vi "FPGA_MotorControl.vi"() -> ()   [LabVIEW 2013]
uses:
  <vilib>/Platform/TimedLoop/XDataNode/timing_clust.ctl
  <vilib>/Platform/TimedLoop/XDataNode/nitl_modes.ctl
  <vilib>/Platform/TimedLoop/XDataNode/wakeup.ctl
  <vilib>/rvi/FXPMathLib/FxpDiv/subVIs/nifxpmath_Div_SimConfig.ctl
  <vilib>/rvi/Emulation/niFpgaSctlEmulationGetInTimedLoop.vi
  <vilib>/rvi/Emulation/niFpgaEmulationReportErrorSimple.vi
  <vilib>/rvi/Emulation/niFpgaGetClockAttributes.vi
  <vilib>/rvi/Emulation/niFpgaCriticalErrorInLSC.vi
  GVEncoder.vi
  <vilib>/rvi/eio/common/nirviEmuTemplateMethod_errors.vi
  <vilib>/rvi/Emulation/niFpgaProcessEmulError.vi
  <vilib>/rvi/FXPMathLib/FxpDiv/simVIs/DllFxpDivTemp_sub.vi
  <vilib>/Platform/TimedLoop/XDataNode/XDataNode.xnode
  <vilib>/eio/EIONode/EIONode.xnode
  <vilib>/rvi/FXPMathLib/FxpMul/XNode/nifxpmath_Multiplier.xnode
  <vilib>/rvi/FXPMathLib/FxpDiv/XNode/nifxpmath_Div.xnode
  <vilib>/rvi/Analysis/measure/butterworth/XNode/niFpgaButterworthFilter.xnode
  <vilib>/Platform/TimedLoop/XDataNode/XDNodeRunTimeDep.lvlib
  <vilib>/rvi/FXPMathLib/sim/FxpSim.dll
panel:
  in  "Reset Position 8":bool
  in  "Reset Position 7":bool
  in  "Reset Position 6":bool
  in  "Reset Position 5":bool
  in  "Reset Position 4":bool
  out "EncdSpeed":sgl[](array[numeric])
  out "EncdAngle":sgl[](array[numeric]) format="%#.3f"
  in  "2pi":fxp<+/-,32,10>=6.283185243606567 format="%#_39g"
  in  "EncoderCount":fxp<+,16,16>=2048.0
  in  "Reset Position 3":bool
  in  "Reset Position 2":bool
  in  "Reset Position 1":bool
  in  "AO_Value":sgl[](array[numeric])=[0.0, 0.0, 0.0, 0.0, 0.0, 0.0, 0.0, 0.0]
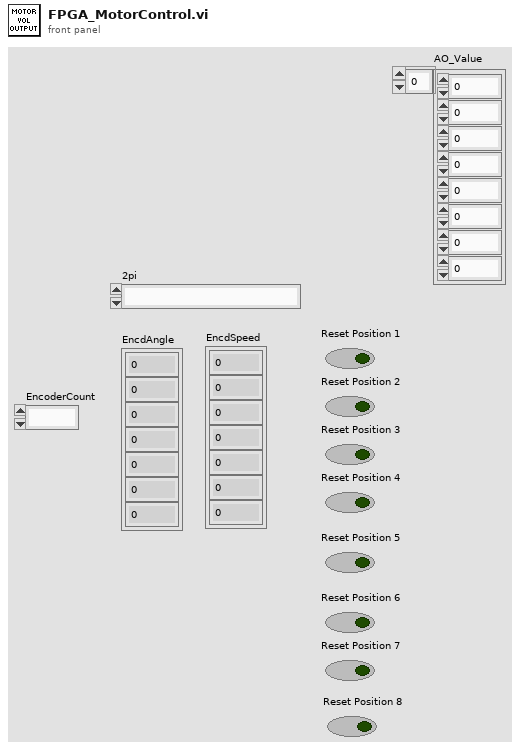
[diagram p1: front panel]
types:
  T1 = typedef "XDNodeRunTimeDep.lvlib/timing_clust.ctl" = cluster{"Expected End [f-1]":u64, "Actual End [f-1]":u64, "Finished Late? [f-1]":bool, "Expected End [i-1]":u64, "Actual End [i-1]":u64, "Finished Late? [i-1]":bool, "Expected Start [i]":u64, "Actual Start [i]":u64, "Expected Start [f]":u64, "Actual Start [f]":u64, "Source Name":string, "Structure Name":string, "Period":i64, "Deadline":i64, "Offset":i64, "Start":i64, "Priority":i32, "Timeout":i32, "Mode":T2, "Wakeup Reason":T3, "Error":errorcluster, "Source Type":string, "Secondary Source Type":string, "Global End Time":u64, "Global Start Time":u64, "Frame Duration":u64, "Iteration Duration":u64, "Assigned CPU":i32, "I/O Scan Engine Mode":u32}
  T2 = typedef "XDNodeRunTimeDep.lvlib/nitl_modes.ctl" = enum32{"No Change", "Process missed periods, maintain original phase", "Discard missed periods, maintain original phase", "Process missed periods, ignore original phase", "Discard missed periods, ignore original phase"}
  T3 = typedef "XDNodeRunTimeDep.lvlib/wakeup.ctl" = enum32{"Normal", "Aborted", "Asynchronous wakeup", "Timing source error", "Timed loop error", "Timeout"}
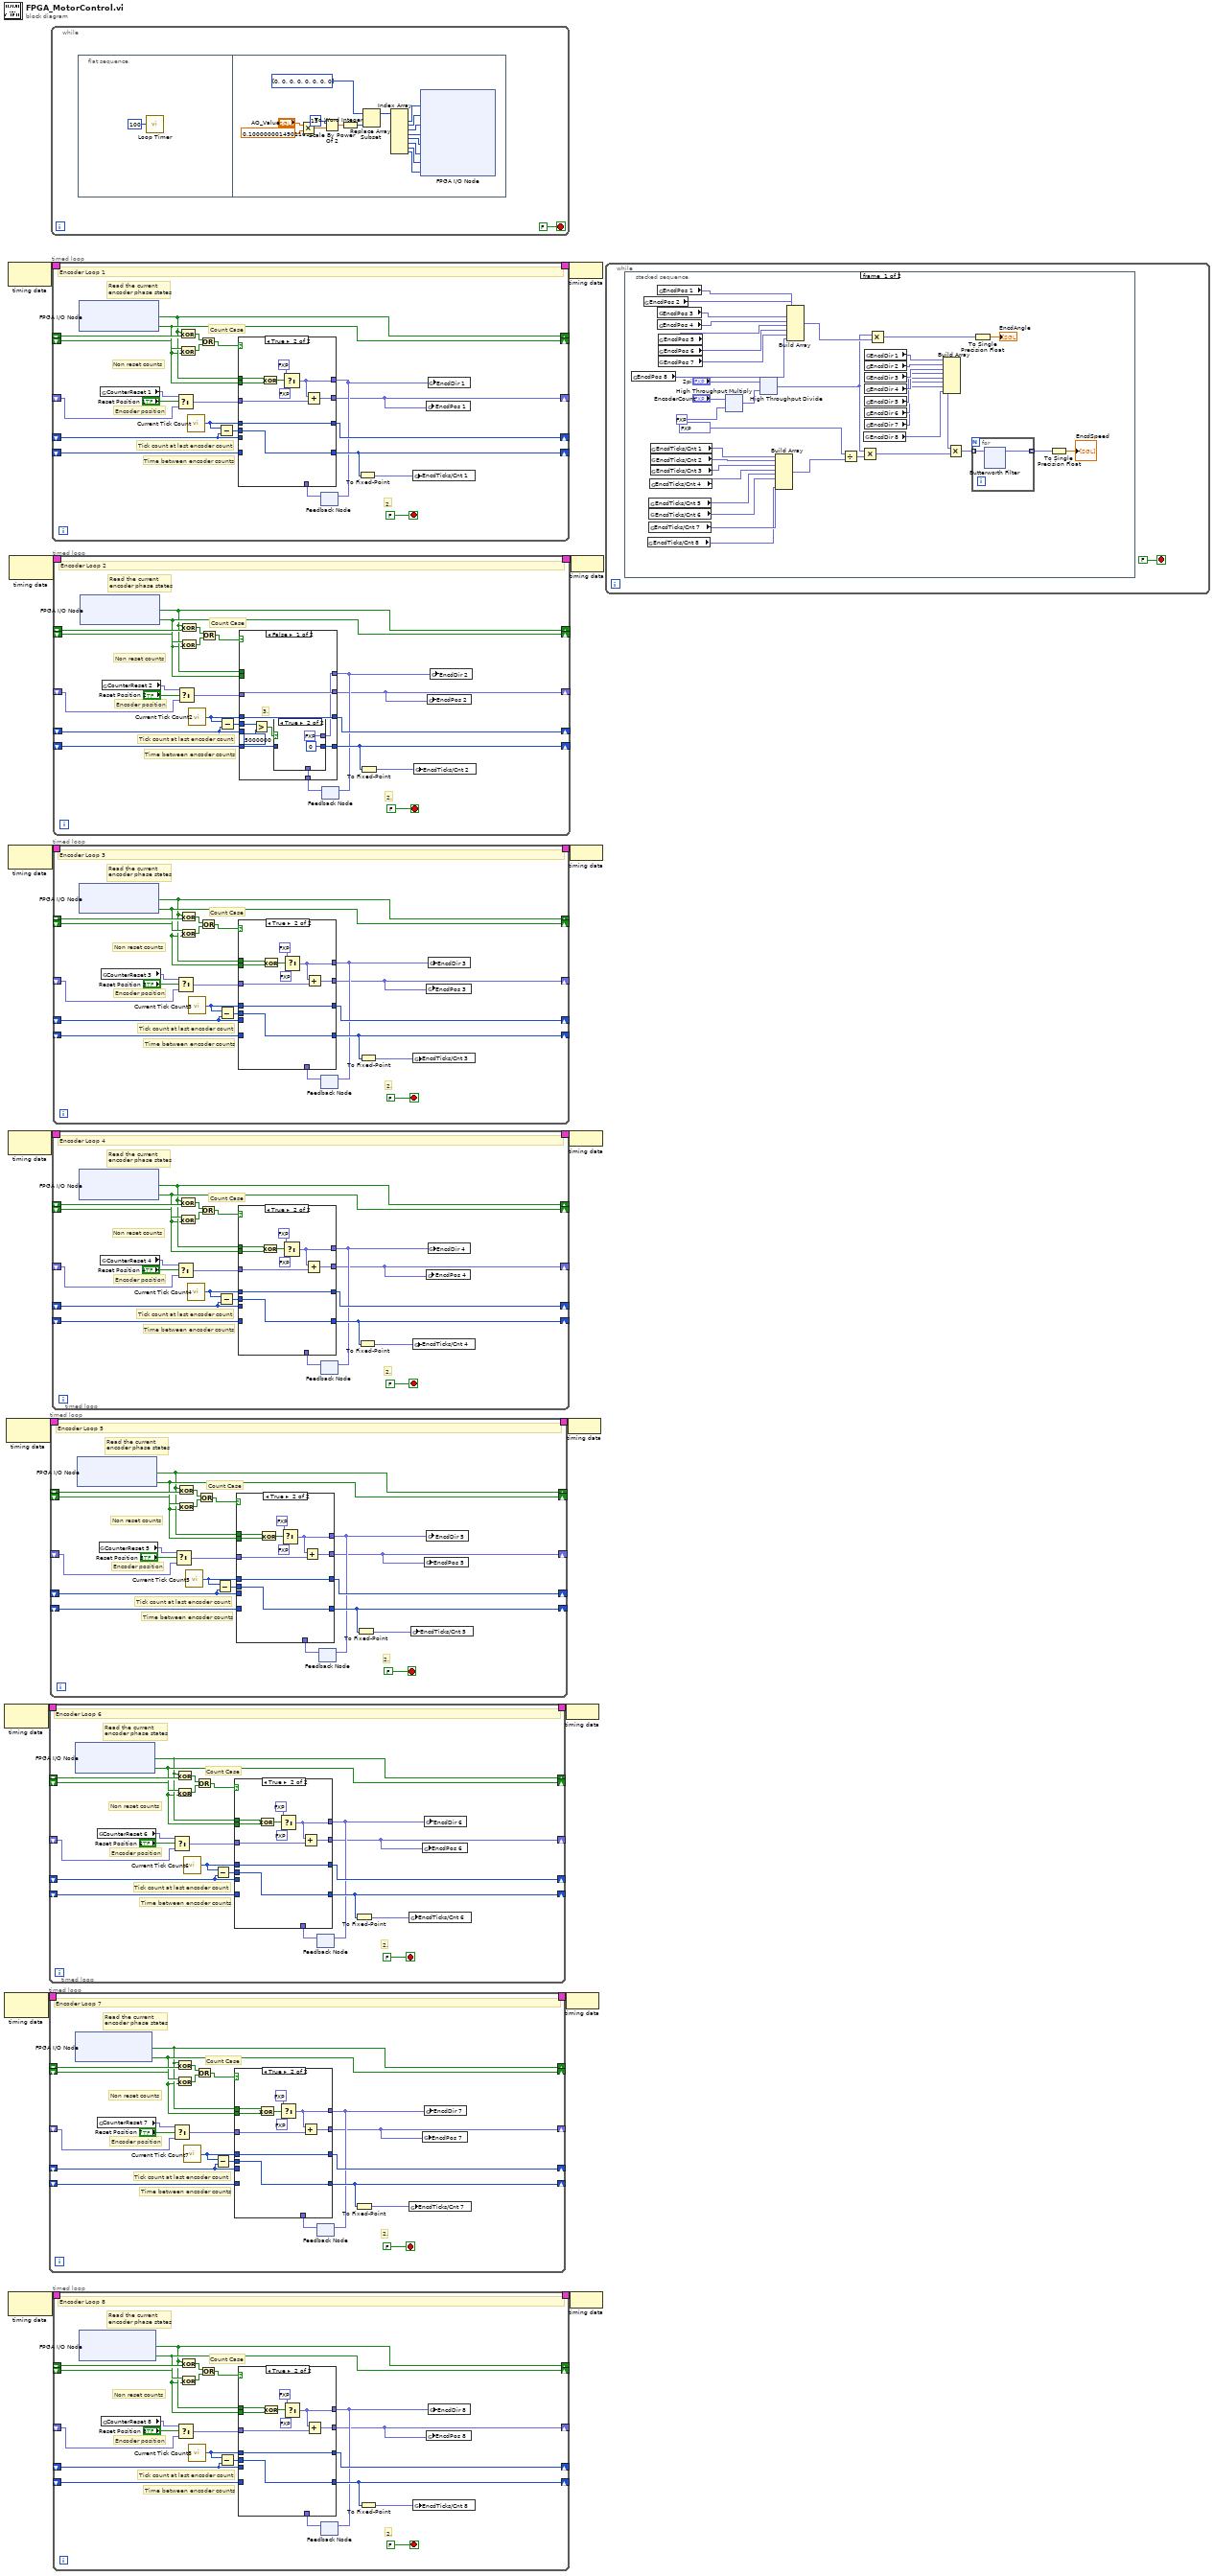
[diagram p0: block diagram]
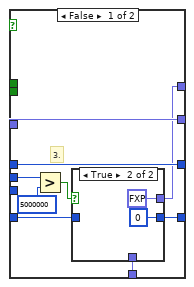
[diagram p2: hidden frame]
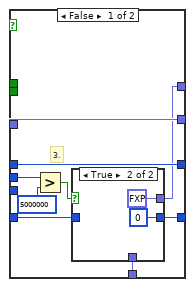
[diagram p4: hidden frame]
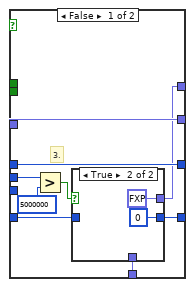
[diagram p6: hidden frame]
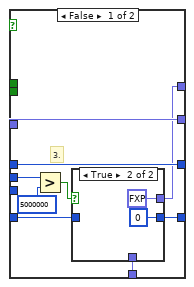
[diagram p8: hidden frame]
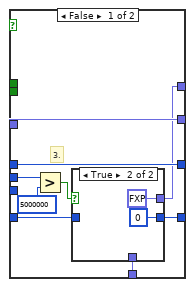
[diagram p10: hidden frame]
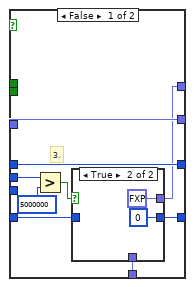
[diagram p12: hidden frame]
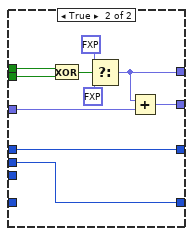
[diagram p15: hidden frame]
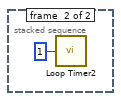
[diagram p16: hidden frame]
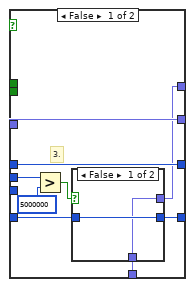
[diagram p17: hidden frame]
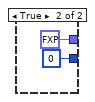
[diagram p18: hidden frame]
diagram:
  n1 = node-c288() -> (w6:T1)  [unwired: 1 in]
  n2 = node-c288() -> (w4:T1)  [unwired: 1 in]
  n3 = node-c288() -> (w8:T1)  [unwired: 1 in]
  n4 = node-c288() -> (w16:T1)  [unwired: 1 in]
  n5 = node-c288() -> (w10:T1)  [unwired: 1 in]
  n6 = node-c288() -> (w12:T1)  [unwired: 1 in]
  n7 = node-c288() -> (w2:T1)  [unwired: 1 in]
  n8 = node-c288() -> (w14:T1)  [unwired: 1 in]
  n9 = timed-loop {
    shift-right: [w32] -> _
    shift-left: _ -> [w38]
    shift-right: [w33] -> _
    shift-left: _ -> [w31]
    shift-right: [w18] -> _
    shift-left: _ -> [w37]
    shift-right: [w36] -> _
    shift-left: _ -> [w30]
    shift-right: [w23] -> _
    shift-left: _ -> [w35]
    timing: w6 -> [_]
    timing-out: [_] -> w5
    stop <- FALSE stop-if-true
    # "Count Case"
    # "2."
    # "Read the current\nencoder phase states"
    # "Non reset counts"
    # "Encoder position"
    # "Time between encoder counts"
    # "Tick count at last encoder count"
    # "Encoder Loop 6"
    n10 = xnode "FPGA I/O Node"() -> ("Connector1/DIO22"=w32:bool, "Connector1/DIO21"=w33:bool)  [unwired: 2 in, 2 out]
    n11 = global read "GVEncoder.vi" "CounterReset 6"() -> (w19:fxp<+/-,32,32>)
    n12 = Select(t=w19, s="Reset Position 6", f=w37) -> (s? t:f=w26:fxp<+/-,32,32>)
    n13 = Exclusive Or(1:w38, 2:w32) -> (0:w29:bool)
    n14 = Exclusive Or(1:w31, 2:w33) -> (0:w28:bool)
    n15 = call "Current Tick Count6"() -> ("Tick Count(Ticks)"=w24:u32)
    n16 = Or(x=w29, y=w28) -> (x .or. y?=w27:bool)
    n17 = Subtract(x=w24, y=w30) -> (x-y=w25:u32)
    n18 = feedback #1() -> (w21:fxp<+/-,2,2>)  [unwired: 1 in]
    n19 = case shown="True" w27 {
      tunnel: [w47 w55] -> w18
      tunnel: w26 -> [w47 w61]
      tunnel: [w41 w54] -> w36
      tunnel: w30 -> [w41 _]
      tunnel: [w44 w53] -> w23
      tunnel: w35 -> [w43 _]
      tunnel: w32 -> [_ w57]
      tunnel: w31 -> [_ w56]
      tunnel: w25 -> [w42 w53]
      tunnel: w24 -> [_ w54]
      tunnel: [w40 w52] -> w20
      tunnel: w21 -> [w39 _]
      frame False {
        # "3."
        n20 = Greater?(x=w42, y=u32 5000000 ("x")) -> (0:w45:bool)
        n21 = case shown="True" w45 {
          tunnel: [w49 u32 0 ("x")] -> w44
          tunnel: w43 -> [w49 _]
          tunnel: [w48 fxp<+/-,2,2> 0.0 ("16 bit")] -> w40
          tunnel: w39 -> [w48 _]
          frame False {
          }
          frame True {
          }
        }
      }
      frame True {
        n22 = Exclusive Or(1:w56, 2:w57) -> (0:w58:bool)
        n23 = Select(t=fxp<+,1,1> 1.0 ("16 bit"), s=w58, f=fxp<+/-,1,1> -1.0 ("16 bit")) -> (s? t:f=w52:fxp<+/-,2,2>)
        n24 = Add(x=w52, y=w61) -> (x+y=w55:fxp<+/-,32,32>)
      }
    }
    n25 = feedback-in #1(w20) -> ()
    n26 = To Fixed-Point(number=w23) -> (fixed-point=w17:fxp<+,32,32>)  [unwired: 1 in]
    n27 = global write "GVEncoder.vi" "EncdTicks/Cnt 6"(w17) -> ()
    n28 = global write "GVEncoder.vi" "EncdPos 6"(w18) -> ()
    n29 = global write "GVEncoder.vi" "EncdDir 6"(w20) -> ()
  }
  n30 = timed-loop {
    shift-right: [w79] -> _
    shift-left: _ -> [w85]
    shift-right: [w80] -> _
    shift-left: _ -> [w78]
    shift-right: [w65] -> _
    shift-left: _ -> [w84]
    shift-right: [w83] -> _
    shift-left: _ -> [w77]
    shift-right: [w70] -> _
    shift-left: _ -> [w82]
    timing: w4 -> [_]
    timing-out: [_] -> w3
    stop <- FALSE stop-if-true
    # "Count Case"
    # "2."
    # "Read the current\nencoder phase states"
    # "Non reset counts"
    # "Encoder position"
    # "Time between encoder counts"
    # "Tick count at last encoder count"
    # "Encoder Loop 7"
    n31 = xnode "FPGA I/O Node"() -> ("Connector1/DIO0"=w79:bool, "Connector1/DIO1"=w80:bool)  [unwired: 2 in, 2 out]
    n32 = global read "GVEncoder.vi" "CounterReset 7"() -> (w66:fxp<+/-,32,32>)
    n33 = Select(t=w66, s="Reset Position 7", f=w84) -> (s? t:f=w73:fxp<+/-,32,32>)
    n34 = Exclusive Or(1:w85, 2:w79) -> (0:w76:bool)
    n35 = Exclusive Or(1:w78, 2:w80) -> (0:w75:bool)
    n36 = call "Current Tick Count7"() -> ("Tick Count(Ticks)"=w71:u32)
    n37 = Or(x=w76, y=w75) -> (x .or. y?=w74:bool)
    n38 = Subtract(x=w71, y=w77) -> (x-y=w72:u32)
    n39 = feedback #2() -> (w68:fxp<+/-,2,2>)  [unwired: 1 in]
    n40 = case shown="True" w74 {
      tunnel: [w94 w102] -> w65
      tunnel: w73 -> [w94 w108]
      tunnel: [w88 w101] -> w83
      tunnel: w77 -> [w88 _]
      tunnel: [w91 w100] -> w70
      tunnel: w82 -> [w90 _]
      tunnel: w79 -> [_ w104]
      tunnel: w78 -> [_ w103]
      tunnel: w72 -> [w89 w100]
      tunnel: w71 -> [_ w101]
      tunnel: [w87 w99] -> w67
      tunnel: w68 -> [w86 _]
      frame False {
        # "3."
        n41 = Greater?(x=w89, y=u32 5000000 ("x")) -> (0:w92:bool)
        n42 = case shown="True" w92 {
          tunnel: [w96 u32 0 ("x")] -> w91
          tunnel: w90 -> [w96 _]
          tunnel: [w95 fxp<+/-,2,2> 0.0 ("16 bit")] -> w87
          tunnel: w86 -> [w95 _]
          frame False {
          }
          frame True {
          }
        }
      }
      frame True {
        n43 = Exclusive Or(1:w103, 2:w104) -> (0:w105:bool)
        n44 = Select(t=fxp<+,1,1> 1.0 ("16 bit"), s=w105, f=fxp<+/-,1,1> -1.0 ("16 bit")) -> (s? t:f=w99:fxp<+/-,2,2>)
        n45 = Add(x=w99, y=w108) -> (x+y=w102:fxp<+/-,32,32>)
      }
    }
    n46 = feedback-in #2(w67) -> ()
    n47 = To Fixed-Point(number=w70) -> (fixed-point=w64:fxp<+,32,32>)  [unwired: 1 in]
    n48 = global write "GVEncoder.vi" "EncdTicks/Cnt 7"(w64) -> ()
    n49 = global write "GVEncoder.vi" "EncdPos 7"(w65) -> ()
    n50 = global write "GVEncoder.vi" "EncdDir 7"(w67) -> ()
  }
  n51 = timed-loop {
    shift-right: [w126] -> _
    shift-left: _ -> [w132]
    shift-right: [w127] -> _
    shift-left: _ -> [w125]
    shift-right: [w112] -> _
    shift-left: _ -> [w131]
    shift-right: [w130] -> _
    shift-left: _ -> [w124]
    shift-right: [w117] -> _
    shift-left: _ -> [w129]
    timing: w8 -> [_]
    timing-out: [_] -> w7
    stop <- FALSE stop-if-true
    # "Count Case"
    # "2."
    # "Read the current\nencoder phase states"
    # "Non reset counts"
    # "Encoder position"
    # "Time between encoder counts"
    # "Tick count at last encoder count"
    # "Encoder Loop 5"
    n52 = xnode "FPGA I/O Node"() -> ("Connector1/DIO23"=w126:bool, "Connector1/DIO24"=w127:bool)  [unwired: 2 in, 2 out]
    n53 = global read "GVEncoder.vi" "CounterReset 5"() -> (w113:fxp<+/-,32,32>)
    n54 = Select(t=w113, s="Reset Position 5", f=w131) -> (s? t:f=w120:fxp<+/-,32,32>)
    n55 = Exclusive Or(1:w132, 2:w126) -> (0:w123:bool)
    n56 = Exclusive Or(1:w125, 2:w127) -> (0:w122:bool)
    n57 = call "Current Tick Count5"() -> ("Tick Count(Ticks)"=w118:u32)
    n58 = Or(x=w123, y=w122) -> (x .or. y?=w121:bool)
    n59 = Subtract(x=w118, y=w124) -> (x-y=w119:u32)
    n60 = feedback #3() -> (w115:fxp<+/-,2,2>)  [unwired: 1 in]
    n61 = case shown="True" w121 {
      tunnel: [w141 w149] -> w112
      tunnel: w120 -> [w141 w155]
      tunnel: [w135 w148] -> w130
      tunnel: w124 -> [w135 _]
      tunnel: [w138 w147] -> w117
      tunnel: w129 -> [w137 _]
      tunnel: w126 -> [_ w151]
      tunnel: w125 -> [_ w150]
      tunnel: w119 -> [w136 w147]
      tunnel: w118 -> [_ w148]
      tunnel: [w134 w146] -> w114
      tunnel: w115 -> [w133 _]
      frame False {
        # "3."
        n62 = Greater?(x=w136, y=u32 5000000 ("x")) -> (0:w139:bool)
        n63 = case shown="True" w139 {
          tunnel: [w143 u32 0 ("x")] -> w138
          tunnel: w137 -> [w143 _]
          tunnel: [w142 fxp<+/-,2,2> 0.0 ("16 bit")] -> w134
          tunnel: w133 -> [w142 _]
          frame False {
          }
          frame True {
          }
        }
      }
      frame True {
        n64 = Exclusive Or(1:w150, 2:w151) -> (0:w152:bool)
        n65 = Select(t=fxp<+,1,1> 1.0 ("16 bit"), s=w152, f=fxp<+/-,1,1> -1.0 ("16 bit")) -> (s? t:f=w146:fxp<+/-,2,2>)
        n66 = Add(x=w146, y=w155) -> (x+y=w149:fxp<+/-,32,32>)
      }
    }
    n67 = feedback-in #3(w114) -> ()
    n68 = To Fixed-Point(number=w117) -> (fixed-point=w111:fxp<+,32,32>)  [unwired: 1 in]
    n69 = global write "GVEncoder.vi" "EncdTicks/Cnt 5"(w111) -> ()
    n70 = global write "GVEncoder.vi" "EncdPos 5"(w112) -> ()
    n71 = global write "GVEncoder.vi" "EncdDir 5"(w114) -> ()
  }
  n72 = while {
    stop <- FALSE stop-if-true
    n73 = flat-sequence {
      frame #0 {
        n74 = call "Loop Timer"("Count(uSec)"=u32 100) -> ()  [unwired: 1 out]
      }
      frame #1 {
        n75 = Multiply(x="AO_Value", y=sgl 0.1 ("Numeric")) -> (x*y=w172:sgl[])
        n76 = Scale By Power Of 2(n=i16 15, x=w172) -> (x*2^n=w171:sgl[])
        n77 = To Word Integer(number=w171) -> (16bit integer=w162:i16[])
        n78 = Replace Array Subset(array=i16[] [0, 0, 0, 0, 0, 0, 0, 0], new element=w162) -> (w161:i16[])  [unwired: 1 in]
        n79 = Index Array(array=w161) -> (element #1=w170:i16, element #2=w169:i16, element #3=w168:i16, element #4=w167:i16, element #5=w166:i16, element #6=w165:i16, element #7=w164:i16, element #8=w163:i16)  [unwired: 8 in]
        n80 = xnode "FPGA I/O Node"("Connector0/AO0"=w170, "Connector0/AO1"=w169, "Connector0/AO2"=w168, "Connector0/AO3"=w167, "Connector0/AO4"=w166, "Connector0/AO5"=w165, "Connector0/AO6"=w164, "Connector0/AO7"=w163) -> ()  [unwired: 8 in, 8 out]
      }
    }
  }
  n81 = timed-loop {
    shift-right: [w191] -> _
    shift-left: _ -> [w197]
    shift-right: [w192] -> _
    shift-left: _ -> [w190]
    shift-right: [w177] -> _
    shift-left: _ -> [w196]
    shift-right: [w195] -> _
    shift-left: _ -> [w189]
    shift-right: [w182] -> _
    shift-left: _ -> [w194]
    timing: w16 -> [_]
    timing-out: [_] -> w15
    stop <- FALSE stop-if-true
    # "Count Case"
    # "2."
    # "Read the current\nencoder phase states"
    # "Non reset counts"
    # "Encoder position"
    # "Time between encoder counts"
    # "Tick count at last encoder count"
    # "Encoder Loop 1"
    n82 = xnode "FPGA I/O Node"() -> ("Connector1/DIO13"=w191:bool, "Connector1/DIO12"=w192:bool)  [unwired: 2 in, 2 out]
    n83 = global read "GVEncoder.vi" "CounterReset 1"() -> (w178:fxp<+/-,32,32>)
    n84 = Select(t=w178, s="Reset Position 1", f=w196) -> (s? t:f=w185:fxp<+/-,32,32>)
    n85 = Exclusive Or(1:w197, 2:w191) -> (0:w188:bool)
    n86 = Exclusive Or(1:w190, 2:w192) -> (0:w187:bool)
    n87 = call "Current Tick Count"() -> ("Tick Count(Ticks)"=w183:u32)
    n88 = Or(x=w188, y=w187) -> (x .or. y?=w186:bool)
    n89 = Subtract(x=w183, y=w189) -> (x-y=w184:u32)
    n90 = feedback #4() -> (w180:fxp<+/-,2,2>)  [unwired: 1 in]
    n91 = case shown="True" w186 {
      tunnel: [w206 w214] -> w177
      tunnel: w185 -> [w206 w220]
      tunnel: [w200 w213] -> w195
      tunnel: w189 -> [w200 _]
      tunnel: [w203 w212] -> w182
      tunnel: w194 -> [w202 _]
      tunnel: w191 -> [_ w216]
      tunnel: w190 -> [_ w215]
      tunnel: w184 -> [w201 w212]
      tunnel: w183 -> [_ w213]
      tunnel: [w199 w211] -> w179
      tunnel: w180 -> [w198 _]
      frame False {
        # "3."
        n92 = Greater?(x=w201, y=u32 5000000 ("x")) -> (0:w204:bool)
        n93 = case shown="False" w204 {
          tunnel: [w208 u32 0 ("x")] -> w203
          tunnel: w202 -> [w208 _]
          tunnel: [w207 fxp<+/-,2,2> 0.0 ("16 bit")] -> w199
          tunnel: w198 -> [w207 _]
          frame False {
          }
          frame True {
          }
        }
      }
      frame True {
        n94 = Exclusive Or(1:w215, 2:w216) -> (0:w217:bool)
        n95 = Select(t=fxp<+,1,1> 1.0 ("16 bit"), s=w217, f=fxp<+/-,1,1> -1.0 ("16 bit")) -> (s? t:f=w211:fxp<+/-,2,2>)
        n96 = Add(x=w211, y=w220) -> (x+y=w214:fxp<+/-,32,32>)
      }
    }
    n97 = feedback-in #4(w179) -> ()
    n98 = To Fixed-Point(number=w182) -> (fixed-point=w176:fxp<+,32,32>)  [unwired: 1 in]
    n99 = global write "GVEncoder.vi" "EncdTicks/Cnt 1"(w176) -> ()
    n100 = global write "GVEncoder.vi" "EncdPos 1"(w177) -> ()
    n101 = global write "GVEncoder.vi" "EncdDir 1"(w179) -> ()
  }
  n102 = timed-loop {
    shift-right: [w238] -> _
    shift-left: _ -> [w244]
    shift-right: [w239] -> _
    shift-left: _ -> [w237]
    shift-right: [w224] -> _
    shift-left: _ -> [w243]
    shift-right: [w242] -> _
    shift-left: _ -> [w236]
    shift-right: [w229] -> _
    shift-left: _ -> [w241]
    timing: w10 -> [_]
    timing-out: [_] -> w9
    stop <- FALSE stop-if-true
    # "Count Case"
    # "2."
    # "Read the current\nencoder phase states"
    # "Non reset counts"
    # "Encoder position"
    # "Time between encoder counts"
    # "Tick count at last encoder count"
    # "Encoder Loop 4"
    n103 = xnode "FPGA I/O Node"() -> ("Connector1/DIO19"=w238:bool, "Connector1/DIO18"=w239:bool)  [unwired: 2 in, 2 out]
    n104 = global read "GVEncoder.vi" "CounterReset 4"() -> (w225:fxp<+/-,32,32>)
    n105 = Select(t=w225, s="Reset Position 4", f=w243) -> (s? t:f=w232:fxp<+/-,32,32>)
    n106 = Exclusive Or(1:w244, 2:w238) -> (0:w235:bool)
    n107 = Exclusive Or(1:w237, 2:w239) -> (0:w234:bool)
    n108 = call "Current Tick Count4"() -> ("Tick Count(Ticks)"=w230:u32)
    n109 = Or(x=w235, y=w234) -> (x .or. y?=w233:bool)
    n110 = Subtract(x=w230, y=w236) -> (x-y=w231:u32)
    n111 = feedback #5() -> (w227:fxp<+/-,2,2>)  [unwired: 1 in]
    n112 = case shown="True" w233 {
      tunnel: [w253 w261] -> w224
      tunnel: w232 -> [w253 w267]
      tunnel: [w247 w260] -> w242
      tunnel: w236 -> [w247 _]
      tunnel: [w250 w259] -> w229
      tunnel: w241 -> [w249 _]
      tunnel: w238 -> [_ w263]
      tunnel: w237 -> [_ w262]
      tunnel: w231 -> [w248 w259]
      tunnel: w230 -> [_ w260]
      tunnel: [w246 w258] -> w226
      tunnel: w227 -> [w245 _]
      frame False {
        # "3."
        n113 = Greater?(x=w248, y=u32 5000000 ("x")) -> (0:w251:bool)
        n114 = case shown="True" w251 {
          tunnel: [w255 u32 0 ("x")] -> w250
          tunnel: w249 -> [w255 _]
          tunnel: [w254 fxp<+/-,2,2> 0.0 ("16 bit")] -> w246
          tunnel: w245 -> [w254 _]
          frame False {
          }
          frame True {
          }
        }
      }
      frame True {
        n115 = Exclusive Or(1:w262, 2:w263) -> (0:w264:bool)
        n116 = Select(t=fxp<+,1,1> 1.0 ("16 bit"), s=w264, f=fxp<+/-,1,1> -1.0 ("16 bit")) -> (s? t:f=w258:fxp<+/-,2,2>)
        n117 = Add(x=w258, y=w267) -> (x+y=w261:fxp<+/-,32,32>)
      }
    }
    n118 = feedback-in #5(w226) -> ()
    n119 = To Fixed-Point(number=w229) -> (fixed-point=w223:fxp<+,32,32>)  [unwired: 1 in]
    n120 = global write "GVEncoder.vi" "EncdTicks/Cnt 4"(w223) -> ()
    n121 = global write "GVEncoder.vi" "EncdPos 4"(w224) -> ()
    n122 = global write "GVEncoder.vi" "EncdDir 4"(w226) -> ()
  }
  n123 = timed-loop {
    shift-right: [w285] -> _
    shift-left: _ -> [w291]
    shift-right: [w286] -> _
    shift-left: _ -> [w284]
    shift-right: [w271] -> _
    shift-left: _ -> [w290]
    shift-right: [w289] -> _
    shift-left: _ -> [w283]
    shift-right: [w276] -> _
    shift-left: _ -> [w288]
    timing: w12 -> [_]
    timing-out: [_] -> w11
    stop <- FALSE stop-if-true
    # "Count Case"
    # "2."
    # "Read the current\nencoder phase states"
    # "Non reset counts"
    # "Encoder position"
    # "Time between encoder counts"
    # "Tick count at last encoder count"
    # "Encoder Loop 3"
    n124 = xnode "FPGA I/O Node"() -> ("Connector1/DIO16"=w285:bool, "Connector1/DIO15"=w286:bool)  [unwired: 2 in, 2 out]
    n125 = global read "GVEncoder.vi" "CounterReset 3"() -> (w272:fxp<+/-,32,32>)
    n126 = Select(t=w272, s="Reset Position 3", f=w290) -> (s? t:f=w279:fxp<+/-,32,32>)
    n127 = Exclusive Or(1:w291, 2:w285) -> (0:w282:bool)
    n128 = Exclusive Or(1:w284, 2:w286) -> (0:w281:bool)
    n129 = call "Current Tick Count3"() -> ("Tick Count(Ticks)"=w277:u32)
    n130 = Or(x=w282, y=w281) -> (x .or. y?=w280:bool)
    n131 = Subtract(x=w277, y=w283) -> (x-y=w278:u32)
    n132 = feedback #6() -> (w274:fxp<+/-,2,2>)  [unwired: 1 in]
    n133 = case shown="True" w280 {
      tunnel: [w300 w308] -> w271
      tunnel: w279 -> [w300 w314]
      tunnel: [w294 w307] -> w289
      tunnel: w283 -> [w294 _]
      tunnel: [w297 w306] -> w276
      tunnel: w288 -> [w296 _]
      tunnel: w285 -> [_ w310]
      tunnel: w284 -> [_ w309]
      tunnel: w278 -> [w295 w306]
      tunnel: w277 -> [_ w307]
      tunnel: [w293 w305] -> w273
      tunnel: w274 -> [w292 _]
      frame False {
        # "3."
        n134 = Greater?(x=w295, y=u32 5000000 ("x")) -> (0:w298:bool)
        n135 = case shown="True" w298 {
          tunnel: [w302 u32 0 ("x")] -> w297
          tunnel: w296 -> [w302 _]
          tunnel: [w301 fxp<+/-,2,2> 0.0 ("16 bit")] -> w293
          tunnel: w292 -> [w301 _]
          frame False {
          }
          frame True {
          }
        }
      }
      frame True {
        n136 = Exclusive Or(1:w309, 2:w310) -> (0:w311:bool)
        n137 = Select(t=fxp<+,1,1> 1.0 ("16 bit"), s=w311, f=fxp<+/-,1,1> -1.0 ("16 bit")) -> (s? t:f=w305:fxp<+/-,2,2>)
        n138 = Add(x=w305, y=w314) -> (x+y=w308:fxp<+/-,32,32>)
      }
    }
    n139 = feedback-in #6(w273) -> ()
    n140 = To Fixed-Point(number=w276) -> (fixed-point=w270:fxp<+,32,32>)  [unwired: 1 in]
    n141 = global write "GVEncoder.vi" "EncdTicks/Cnt 3"(w270) -> ()
    n142 = global write "GVEncoder.vi" "EncdPos 3"(w271) -> ()
    n143 = global write "GVEncoder.vi" "EncdDir 3"(w273) -> ()
  }
  n144 = timed-loop {
    shift-right: [w332] -> _
    shift-left: _ -> [w338]
    shift-right: [w333] -> _
    shift-left: _ -> [w331]
    shift-right: [w318] -> _
    shift-left: _ -> [w337]
    shift-right: [w336] -> _
    shift-left: _ -> [w330]
    shift-right: [w323] -> _
    shift-left: _ -> [w335]
    timing: w2 -> [_]
    timing-out: [_] -> w1
    stop <- FALSE stop-if-true
    # "Count Case"
    # "2."
    # "Read the current\nencoder phase states"
    # "Non reset counts"
    # "Encoder position"
    # "Time between encoder counts"
    # "Tick count at last encoder count"
    # "Encoder Loop 8"
    n145 = xnode "FPGA I/O Node"() -> ("Connector1/DIO3"=w332:bool, "Connector1/DIO4"=w333:bool)  [unwired: 2 in, 2 out]
    n146 = global read "GVEncoder.vi" "CounterReset 8"() -> (w319:fxp<+/-,32,32>)
    n147 = Select(t=w319, s="Reset Position 8", f=w337) -> (s? t:f=w326:fxp<+/-,32,32>)
    n148 = Exclusive Or(1:w338, 2:w332) -> (0:w329:bool)
    n149 = Exclusive Or(1:w331, 2:w333) -> (0:w328:bool)
    n150 = call "Current Tick Count8"() -> ("Tick Count(Ticks)"=w324:u32)
    n151 = Or(x=w329, y=w328) -> (x .or. y?=w327:bool)
    n152 = Subtract(x=w324, y=w330) -> (x-y=w325:u32)
    n153 = feedback #7() -> (w321:fxp<+/-,2,2>)  [unwired: 1 in]
    n154 = case shown="True" w327 {
      tunnel: [w347 w355] -> w318
      tunnel: w326 -> [w347 w361]
      tunnel: [w341 w354] -> w336
      tunnel: w330 -> [w341 _]
      tunnel: [w344 w353] -> w323
      tunnel: w335 -> [w343 _]
      tunnel: w332 -> [_ w357]
      tunnel: w331 -> [_ w356]
      tunnel: w325 -> [w342 w353]
      tunnel: w324 -> [_ w354]
      tunnel: [w340 w352] -> w320
      tunnel: w321 -> [w339 _]
      frame False {
        # "3."
        n155 = Greater?(x=w342, y=u32 5000000 ("x")) -> (0:w345:bool)
        n156 = case shown="True" w345 {
          tunnel: [w349 u32 0 ("x")] -> w344
          tunnel: w343 -> [w349 _]
          tunnel: [w348 fxp<+/-,2,2> 0.0 ("16 bit")] -> w340
          tunnel: w339 -> [w348 _]
          frame False {
          }
          frame True {
          }
        }
      }
      frame True {
        n157 = Exclusive Or(1:w356, 2:w357) -> (0:w358:bool)
        n158 = Select(t=fxp<+,1,1> 1.0 ("16 bit"), s=w358, f=fxp<+/-,1,1> -1.0 ("16 bit")) -> (s? t:f=w352:fxp<+/-,2,2>)
        n159 = Add(x=w352, y=w361) -> (x+y=w355:fxp<+/-,32,32>)
      }
    }
    n160 = feedback-in #7(w320) -> ()
    n161 = To Fixed-Point(number=w323) -> (fixed-point=w317:fxp<+,32,32>)  [unwired: 1 in]
    n162 = global write "GVEncoder.vi" "EncdTicks/Cnt 8"(w317) -> ()
    n163 = global write "GVEncoder.vi" "EncdPos 8"(w318) -> ()
    n164 = global write "GVEncoder.vi" "EncdDir 8"(w320) -> ()
  }
  n165 = timed-loop {
    shift-right: [w379] -> _
    shift-left: _ -> [w385]
    shift-right: [w380] -> _
    shift-left: _ -> [w378]
    shift-right: [w365] -> _
    shift-left: _ -> [w384]
    shift-right: [w383] -> _
    shift-left: _ -> [w377]
    shift-right: [w370] -> _
    shift-left: _ -> [w382]
    timing: w14 -> [_]
    timing-out: [_] -> w13
    stop <- FALSE stop-if-true
    # "Count Case"
    # "2."
    # "Read the current\nencoder phase states"
    # "Non reset counts"
    # "Encoder position"
    # "Time between encoder counts"
    # "Tick count at last encoder count"
    # "Encoder Loop 2"
    n166 = xnode "FPGA I/O Node"() -> ("Connector1/DIO29"=w379:bool, "Connector1/DIO31"=w380:bool)  [unwired: 2 in, 2 out]
    n167 = global read "GVEncoder.vi" "CounterReset 2"() -> (w366:fxp<+/-,32,32>)
    n168 = Select(t=w366, s="Reset Position 2", f=w384) -> (s? t:f=w373:fxp<+/-,32,32>)
    n169 = Exclusive Or(1:w385, 2:w379) -> (0:w376:bool)
    n170 = Exclusive Or(1:w378, 2:w380) -> (0:w375:bool)
    n171 = call "Current Tick Count2"() -> ("Tick Count(Ticks)"=w371:u32)
    n172 = Or(x=w376, y=w375) -> (x .or. y?=w374:bool)
    n173 = Subtract(x=w371, y=w377) -> (x-y=w372:u32)
    n174 = feedback #8() -> (w368:fxp<+/-,2,2>)  [unwired: 1 in]
    n175 = case shown="False" w374 {
      tunnel: [w394 w402] -> w365
      tunnel: w373 -> [w394 w408]
      tunnel: [w388 w401] -> w383
      tunnel: w377 -> [w388 _]
      tunnel: [w391 w400] -> w370
      tunnel: w382 -> [w390 _]
      tunnel: w379 -> [_ w404]
      tunnel: w378 -> [_ w403]
      tunnel: w372 -> [w389 w400]
      tunnel: w371 -> [_ w401]
      tunnel: [w387 w399] -> w367
      tunnel: w368 -> [w386 _]
      frame False {
        # "3."
        n176 = Greater?(x=w389, y=u32 5000000 ("x")) -> (0:w392:bool)
        n177 = case shown="True" w392 {
          tunnel: [w396 u32 0 ("x")] -> w391
          tunnel: w390 -> [w396 _]
          tunnel: [w395 fxp<+/-,2,2> 0.0 ("16 bit")] -> w387
          tunnel: w386 -> [w395 _]
          frame False {
          }
          frame True {
          }
        }
      }
      frame True {
        n178 = Exclusive Or(1:w403, 2:w404) -> (0:w405:bool)
        n179 = Select(t=fxp<+,1,1> 1.0 ("16 bit"), s=w405, f=fxp<+/-,1,1> -1.0 ("16 bit")) -> (s? t:f=w399:fxp<+/-,2,2>)
        n180 = Add(x=w399, y=w408) -> (x+y=w402:fxp<+/-,32,32>)
      }
    }
    n181 = feedback-in #8(w367) -> ()
    n182 = To Fixed-Point(number=w370) -> (fixed-point=w364:fxp<+,32,32>)  [unwired: 1 in]
    n183 = global write "GVEncoder.vi" "EncdTicks/Cnt 2"(w364) -> ()
    n184 = global write "GVEncoder.vi" "EncdPos 2"(w365) -> ()
    n185 = global write "GVEncoder.vi" "EncdDir 2"(w367) -> ()
  }
  n186 = node-c288(w5) -> ()
  n187 = node-c288(w3) -> ()
  n188 = node-c288(w7) -> ()
  n189 = node-c288(w15) -> ()
  n190 = node-c288(w9) -> ()
  n191 = node-c288(w11) -> ()
  n192 = node-c288(w1) -> ()
  n193 = node-c288(w13) -> ()
  n194 = while {
    stop <- FALSE stop-if-true
    n195 = stacked-sequence {
      frame #0 {
        n196 = global read "GVEncoder.vi" "EncdPos 8"() -> (w414:fxp<+/-,64,64>)
        n197 = global read "GVEncoder.vi" "EncdPos 2"() -> (w449:fxp<+/-,64,64>)
        n198 = global read "GVEncoder.vi" "EncdTicks/Cnt 8"() -> (w413:fxp<+,32,32>)
        n199 = global read "GVEncoder.vi" "EncdTicks/Cnt 7"() -> (w418:fxp<+,32,32>)
        n200 = global read "GVEncoder.vi" "EncdTicks/Cnt 5"() -> (w420:fxp<+,32,32>)
        n201 = global read "GVEncoder.vi" "EncdTicks/Cnt 6"() -> (w419:fxp<+,32,32>)
        n202 = global read "GVEncoder.vi" "EncdTicks/Cnt 4"() -> (w425:fxp<+,32,32>)
        n203 = global read "GVEncoder.vi" "EncdTicks/Cnt 1"() -> (w443:fxp<+,32,32>)
        n204 = global read "GVEncoder.vi" "EncdTicks/Cnt 2"() -> (w442:fxp<+,32,32>)
        n205 = global read "GVEncoder.vi" "EncdTicks/Cnt 3"() -> (w441:fxp<+,32,32>)
        n206 = global read "GVEncoder.vi" "EncdPos 1"() -> (w450:fxp<+/-,64,64>)
        n207 = global read "GVEncoder.vi" "EncdPos 3"() -> (w448:fxp<+/-,64,64>)
        n208 = global read "GVEncoder.vi" "EncdPos 4"() -> (w426:fxp<+/-,64,64>)
        n209 = global read "GVEncoder.vi" "EncdPos 5"() -> (w423:fxp<+/-,64,64>)
        n210 = global read "GVEncoder.vi" "EncdPos 6"() -> (w422:fxp<+/-,64,64>)
        n211 = global read "GVEncoder.vi" "EncdPos 7"() -> (w421:fxp<+/-,64,64>)
        n212 = xnode "High Throughput Multiply"("x"="EncoderCount", "y"=fxp<+,4,4> 4.0) -> ("x*y"=w428:fxp<+,16,16>)
        n213 = xnode "High Throughput Divide"("x"="2pi", "y"=w428) -> ("x/y"=w431:fxp<+/-,32,4>)
        n214 = Build Array(w443, w442, w441, w425, w420, w419, w418, w413) -> (w439:fxp<+,32,32>[])
        n215 = Build Array(w450, w449, w448, w426, w423, w422, w421, w414) -> (w432:fxp<+/-,64,64>[])
        n216 = Divide(x=fxp<+,32,32> 40000000.0, y=w439) -> (x/y=w437:fxp<+,64,32>[])
        n217 = Multiply(x=w431, y=w437) -> (x*y=w436:fxp<+,32,16>[])
        n218 = global read "GVEncoder.vi" "EncdDir 8"() -> (w412:fxp<+/-,2,2>)
        n219 = global read "GVEncoder.vi" "EncdDir 1"() -> (w446:fxp<+/-,2,2>)
        n220 = global read "GVEncoder.vi" "EncdDir 2"() -> (w445:fxp<+/-,2,2>)
        n221 = global read "GVEncoder.vi" "EncdDir 3"() -> (w444:fxp<+/-,2,2>)
        n222 = global read "GVEncoder.vi" "EncdDir 4"() -> (w424:fxp<+/-,2,2>)
        n223 = global read "GVEncoder.vi" "EncdDir 5"() -> (w417:fxp<+/-,2,2>)
        n224 = global read "GVEncoder.vi" "EncdDir 6"() -> (w416:fxp<+/-,2,2>)
        n225 = global read "GVEncoder.vi" "EncdDir 7"() -> (w415:fxp<+/-,2,2>)
        n226 = Multiply(x=w431, y=w432) -> (x*y=w430:fxp<+/-,64,48>[])
        n227 = Build Array(w446, w445, w444, w424, w417, w416, w415, w412) -> (w440:fxp<+/-,2,2>[])
        n228 = Multiply(x=w440, y=w436) -> (x*y=w434:fxp<+/-,16,4>[])
        n229 = for {
          tunnel: w434 -> [w453] mode=indexing
          tunnel: [w452] -> w433 mode=indexing
          n230 = xnode "Butterworth Filter"("input data"=w453) -> ("output data"=w452:fxp<+/-,20,8>)  [unwired: 2 in, 1 out]
        }
        n231 = To Single Precision Float(number=w430) -> (single precision float=→"EncdAngle":sgl[])
        n232 = To Single Precision Float(number=w433) -> (single precision float=→"EncdSpeed":sgl[])
      }
      frame #1 {
        n233 = call "Loop Timer2"("Count(uSec)"=u32 1) -> ()  [unwired: 1 out]
      }
    }
  }
